vi "SVPO Average Dual-Channel Spectrum Measurements (Complex) with IC.vi"(0 "complex spectrum X":T9 {"spectrum info"."x-axis units" items=["Time (s)"=0, "Frequency-CB (Hz)"=1, "Frequency-CPB (Hz)"=1248, "Frequency-Arbitrary (Hz)"=2357, "Quefrency (s)"=2, "Revolutions (rev)"=3, "Order"=4, "Speed (RPM)"=11, "Speed (rad/s)"=21, "Index"=65535]; "spectrum info"."weighting filter" items=["Linear", "A-weighting", "B-weighting", "C-weighting", "ITU-R 468-4", "Dolby", "CCITT", "C-message", "Wb", "Wc", "Wd", "We", "Wf", "Wh", "Wj", "Wk", "Wm", "AES17 20 kHz lowpass", "AES17 40 kHz lowpass", "AES17 20 kHz highpass", "AES17 40 kHz highpass"]; "spectrum info"."dB reference [EU]" format="%.2f"; "spectrum info"."engineering units" items=["custom..."=0, "V"=1, "A"=21, "C"=30, "pC"=31, "s"=32, "-"=29, "Pa"=2, "N"=20, "g"=3, "m/s^2"=4, "m/s"=5, "m"=6, "mm/s"=12, "mm"=13, "micron/s"=14, "micron"=15, "in/s^2"=7, "in/s"=8, "in"=9, "mil/s"=10, "mil"=11, "rad/s^2"=16, "rad/s"=17, "rad"=18, "deg/s^2"=26, "deg/s"=27, "deg"=28, "RPM"=22, "cycle/s^2"=23, "Hz"=24, "cycle"=25, "strain"=19]; "spectrum info"."spectral info"."window" items=["None "=0, "Hanning"=1, "Hamming"=2, "Blackman-Harris"=3, "Exact Blackman"=4, "Blackman"=5, "Flat Top"=6, "4 Term B-Harris "=7, "7 Term B-Harris"=8, "Low Sidelobe"=9, "Force - Exponential"=10, "Gaussian"=62]}, 1 "complex spectrum Y":T9 {"spectrum info"."x-axis units" items=["Time (s)"=0, "Frequency-CB (Hz)"=1, "Frequency-CPB (Hz)"=1248, "Frequency-Arbitrary (Hz)"=2357, "Quefrency (s)"=2, "Revolutions (rev)"=3, "Order"=4, "Speed (RPM)"=11, "Speed (rad/s)"=21, "Index"=65535]; "spectrum info"."weighting filter" items=["Linear", "A-weighting", "B-weighting", "C-weighting", "ITU-R 468-4", "Dolby", "CCITT", "C-message", "Wb", "Wc", "Wd", "We", "Wf", "Wh", "Wj", "Wk", "Wm", "AES17 20 kHz lowpass", "AES17 40 kHz lowpass", "AES17 20 kHz highpass", "AES17 40 kHz highpass"]; "spectrum info"."dB reference [EU]" format="%.2f"; "spectrum info"."engineering units" items=["custom..."=0, "V"=1, "A"=21, "C"=30, "pC"=31, "s"=32, "-"=29, "Pa"=2, "N"=20, "g"=3, "m/s^2"=4, "m/s"=5, "m"=6, "mm/s"=12, "mm"=13, "micron/s"=14, "micron"=15, "in/s^2"=7, "in/s"=8, "in"=9, "mil/s"=10, "mil"=11, "rad/s^2"=16, "rad/s"=17, "rad"=18, "deg/s^2"=26, "deg/s"=27, "deg"=28, "RPM"=22, "cycle/s^2"=23, "Hz"=24, "cycle"=25, "strain"=19]; "spectrum info"."spectral info"."window" items=["None "=0, "Hanning"=1, "Hamming"=2, "Blackman-Harris"=3, "Exact Blackman"=4, "Blackman"=5, "Flat Top"=6, "4 Term B-Harris "=7, "7 Term B-Harris"=8, "Low Sidelobe"=9, "Force - Exponential"=10, "Gaussian"=62]}, 2 "averaging mode (RMS)":T1(ring)=enum."RMS averaging", 3 "averaging weighting mode (Linear)":enum16{"Linear", "Exponential"}(ring), 5 "initial conditions":T10 {"complex cross"."spectrum info"."x-axis units" items=["Time (s)"=0, "Frequency-CB (Hz)"=1, "Frequency-CPB (Hz)"=1248, "Frequency-Arbitrary (Hz)"=2357, "Quefrency (s)"=2, "Revolutions (rev)"=3, "Order"=4, "Speed (RPM)"=11, "Speed (rad/s)"=21, "Index"=65535]; "complex cross"."spectrum info"."weighting filter" items=["Linear", "A-weighting", "B-weighting", "C-weighting", "ITU-R 468-4", "Dolby", "CCITT", "C-message", "Wb", "Wc", "Wd", "We", "Wf", "Wh", "Wj", "Wk", "Wm", "AES17 20 kHz lowpass", "AES17 40 kHz lowpass", "AES17 20 kHz highpass", "AES17 40 kHz highpass"]; "complex cross"."spectrum info"."dB reference [EU]" format="%.2f"; "complex cross"."spectrum info"."engineering units" items=["custom..."=0, "V"=1, "A"=21, "C"=30, "pC"=31, "s"=32, "-"=29, "Pa"=2, "N"=20, "g"=3, "m/s^2"=4, "m/s"=5, "m"=6, "mm/s"=12, "mm"=13, "micron/s"=14, "micron"=15, "in/s^2"=7, "in/s"=8, "in"=9, "mil/s"=10, "mil"=11, "rad/s^2"=16, "rad/s"=17, "rad"=18, "deg/s^2"=26, "deg/s"=27, "deg"=28, "RPM"=22, "cycle/s^2"=23, "Hz"=24, "cycle"=25, "strain"=19]; "complex cross"."spectrum info"."spectral info"."window" items=["None "=0, "Hanning"=1, "Hamming"=2, "Blackman-Harris"=3, "Exact Blackman"=4, "Blackman"=5, "Flat Top"=6, "4 Term B-Harris "=7, "7 Term B-Harris"=8, "Low Sidelobe"=9, "Force - Exponential"=10, "Gaussian"=62]; "complex X"."spectrum info"."x-axis units" items=["Time (s)"=0, "Frequency-CB (Hz)"=1, "Frequency-CPB (Hz)"=1248, "Frequency-Arbitrary (Hz)"=2357, "Quefrency (s)"=2, "Revolutions (rev)"=3, "Order"=4, "Speed (RPM)"=11, "Speed (rad/s)"=21, "Index"=65535]; "complex X"."spectrum info"."weighting filter" items=["Linear", "A-weighting", "B-weighting", "C-weighting", "ITU-R 468-4", "Dolby", "CCITT", "C-message", "Wb", "Wc", "Wd", "We", "Wf", "Wh", "Wj", "Wk", "Wm", "AES17 20 kHz lowpass", "AES17 40 kHz lowpass", "AES17 20 kHz highpass", "AES17 40 kHz highpass"]; "complex X"."spectrum info"."dB reference [EU]" format="%.2f"; "complex X"."spectrum info"."engineering units" items=["custom..."=0, "V"=1, "A"=21, "C"=30, "pC"=31, "s"=32, "-"=29, "Pa"=2, "N"=20, "g"=3, "m/s^2"=4, "m/s"=5, "m"=6, "mm/s"=12, "mm"=13, "micron/s"=14, "micron"=15, "in/s^2"=7, "in/s"=8, "in"=9, "mil/s"=10, "mil"=11, "rad/s^2"=16, "rad/s"=17, "rad"=18, "deg/s^2"=26, "deg/s"=27, "deg"=28, "RPM"=22, "cycle/s^2"=23, "Hz"=24, "cycle"=25, "strain"=19]; "complex X"."spectrum info"."spectral info"."window" items=["None "=0, "Hanning"=1, "Hamming"=2, "Blackman-Harris"=3, "Exact Blackman"=4, "Blackman"=5, "Flat Top"=6, "4 Term B-Harris "=7, "7 Term B-Harris"=8, "Low Sidelobe"=9, "Force - Exponential"=10, "Gaussian"=62]; "complex Y"."spectrum info"."x-axis units" items=["Time (s)"=0, "Frequency-CB (Hz)"=1, "Frequency-CPB (Hz)"=1248, "Frequency-Arbitrary (Hz)"=2357, "Quefrency (s)"=2, "Revolutions (rev)"=3, "Order"=4, "Speed (RPM)"=11, "Speed (rad/s)"=21, "Index"=65535]; "complex Y"."spectrum info"."weighting filter" items=["Linear", "A-weighting", "B-weighting", "C-weighting", "ITU-R 468-4", "Dolby", "CCITT", "C-message", "Wb", "Wc", "Wd", "We", "Wf", "Wh", "Wj", "Wk", "Wm", "AES17 20 kHz lowpass", "AES17 40 kHz lowpass", "AES17 20 kHz highpass", "AES17 40 kHz highpass"]; "complex Y"."spectrum info"."dB reference [EU]" format="%.2f"; "complex Y"."spectrum info"."engineering units" items=["custom..."=0, "V"=1, "A"=21, "C"=30, "pC"=31, "s"=32, "-"=29, "Pa"=2, "N"=20, "g"=3, "m/s^2"=4, "m/s"=5, "m"=6, "mm/s"=12, "mm"=13, "micron/s"=14, "micron"=15, "in/s^2"=7, "in/s"=8, "in"=9, "mil/s"=10, "mil"=11, "rad/s^2"=16, "rad/s"=17, "rad"=18, "deg/s^2"=26, "deg/s"=27, "deg"=28, "RPM"=22, "cycle/s^2"=23, "Hz"=24, "cycle"=25, "strain"=19]; "complex Y"."spectrum info"."spectral info"."window" items=["None "=0, "Hanning"=1, "Hamming"=2, "Blackman-Harris"=3, "Exact Blackman"=4, "Blackman"=5, "Flat Top"=6, "4 Term B-Harris "=7, "7 Term B-Harris"=8, "Low Sidelobe"=9, "Force - Exponential"=10, "Gaussian"=62]}, 6 "exponential weight (10 %)":dbl=10.0 min=0.0 max=100.0 step=5.0, 8 "measurement (Cross)":T2(ring), 9 "restart averaging (F)":bool) -> (12 "coherence":cluster{"f0":dbl, "df":dbl, "coherence":dbl[]}, 13 "averages completed out":dbl=1.0, 14 "average measurement spectrum out":T9 {"spectrum info"."x-axis units" items=["Time (s)"=0, "Frequency-CB (Hz)"=1, "Frequency-CPB (Hz)"=1248, "Frequency-Arbitrary (Hz)"=2357, "Quefrency (s)"=2, "Revolutions (rev)"=3, "Order"=4, "Speed (RPM)"=11, "Speed (rad/s)"=21, "Index"=65535]; "spectrum info"."weighting filter" items=["Linear", "A-weighting", "B-weighting", "C-weighting", "ITU-R 468-4", "Dolby", "CCITT", "C-message", "Wb", "Wc", "Wd", "We", "Wf", "Wh", "Wj", "Wk", "Wm", "AES17 20 kHz lowpass", "AES17 40 kHz lowpass", "AES17 20 kHz highpass", "AES17 40 kHz highpass"]; "spectrum info"."dB reference [EU]" format="%.2f"; "spectrum info"."engineering units" items=["custom..."=0, "V"=1, "A"=21, "C"=30, "pC"=31, "s"=32, "-"=29, "Pa"=2, "N"=20, "g"=3, "m/s^2"=4, "m/s"=5, "m"=6, "mm/s"=12, "mm"=13, "micron/s"=14, "micron"=15, "in/s^2"=7, "in/s"=8, "in"=9, "mil/s"=10, "mil"=11, "rad/s^2"=16, "rad/s"=17, "rad"=18, "deg/s^2"=26, "deg/s"=27, "deg"=28, "RPM"=22, "cycle/s^2"=23, "Hz"=24, "cycle"=25, "strain"=19]; "spectrum info"."spectral info"."window" items=["None "=0, "Hanning"=1, "Hamming"=2, "Blackman-Harris"=3, "Exact Blackman"=4, "Blackman"=5, "Flat Top"=6, "4 Term B-Harris "=7, "7 Term B-Harris"=8, "Low Sidelobe"=9, "Force - Exponential"=10, "Gaussian"=62]}, 19 "final conditions":T10 {"complex cross"."spectrum info"."x-axis units" items=["Time (s)"=0, "Frequency-CB (Hz)"=1, "Frequency-CPB (Hz)"=1248, "Frequency-Arbitrary (Hz)"=2357, "Quefrency (s)"=2, "Revolutions (rev)"=3, "Order"=4, "Speed (RPM)"=11, "Speed (rad/s)"=21, "Index"=65535]; "complex cross"."spectrum info"."weighting filter" items=["Linear", "A-weighting", "B-weighting", "C-weighting", "ITU-R 468-4", "Dolby", "CCITT", "C-message", "Wb", "Wc", "Wd", "We", "Wf", "Wh", "Wj", "Wk", "Wm", "AES17 20 kHz lowpass", "AES17 40 kHz lowpass", "AES17 20 kHz highpass", "AES17 40 kHz highpass"]; "complex cross"."spectrum info"."dB reference [EU]" format="%.2f"; "complex cross"."spectrum info"."engineering units" items=["custom..."=0, "V"=1, "A"=21, "C"=30, "pC"=31, "s"=32, "-"=29, "Pa"=2, "N"=20, "g"=3, "m/s^2"=4, "m/s"=5, "m"=6, "mm/s"=12, "mm"=13, "micron/s"=14, "micron"=15, "in/s^2"=7, "in/s"=8, "in"=9, "mil/s"=10, "mil"=11, "rad/s^2"=16, "rad/s"=17, "rad"=18, "deg/s^2"=26, "deg/s"=27, "deg"=28, "RPM"=22, "cycle/s^2"=23, "Hz"=24, "cycle"=25, "strain"=19]; "complex cross"."spectrum info"."spectral info"."window" items=["None "=0, "Hanning"=1, "Hamming"=2, "Blackman-Harris"=3, "Exact Blackman"=4, "Blackman"=5, "Flat Top"=6, "4 Term B-Harris "=7, "7 Term B-Harris"=8, "Low Sidelobe"=9, "Force - Exponential"=10, "Gaussian"=62]; "complex X"."spectrum info"."x-axis units" items=["Time (s)"=0, "Frequency-CB (Hz)"=1, "Frequency-CPB (Hz)"=1248, "Frequency-Arbitrary (Hz)"=2357, "Quefrency (s)"=2, "Revolutions (rev)"=3, "Order"=4, "Speed (RPM)"=11, "Speed (rad/s)"=21, "Index"=65535]; "complex X"."spectrum info"."weighting filter" items=["Linear", "A-weighting", "B-weighting", "C-weighting", "ITU-R 468-4", "Dolby", "CCITT", "C-message", "Wb", "Wc", "Wd", "We", "Wf", "Wh", "Wj", "Wk", "Wm", "AES17 20 kHz lowpass", "AES17 40 kHz lowpass", "AES17 20 kHz highpass", "AES17 40 kHz highpass"]; "complex X"."spectrum info"."dB reference [EU]" format="%.2f"; "complex X"."spectrum info"."engineering units" items=["custom..."=0, "V"=1, "A"=21, "C"=30, "pC"=31, "s"=32, "-"=29, "Pa"=2, "N"=20, "g"=3, "m/s^2"=4, "m/s"=5, "m"=6, "mm/s"=12, "mm"=13, "micron/s"=14, "micron"=15, "in/s^2"=7, "in/s"=8, "in"=9, "mil/s"=10, "mil"=11, "rad/s^2"=16, "rad/s"=17, "rad"=18, "deg/s^2"=26, "deg/s"=27, "deg"=28, "RPM"=22, "cycle/s^2"=23, "Hz"=24, "cycle"=25, "strain"=19]; "complex X"."spectrum info"."spectral info"."window" items=["None "=0, "Hanning"=1, "Hamming"=2, "Blackman-Harris"=3, "Exact Blackman"=4, "Blackman"=5, "Flat Top"=6, "4 Term B-Harris "=7, "7 Term B-Harris"=8, "Low Sidelobe"=9, "Force - Exponential"=10, "Gaussian"=62]; "complex Y"."spectrum info"."x-axis units" items=["Time (s)"=0, "Frequency-CB (Hz)"=1, "Frequency-CPB (Hz)"=1248, "Frequency-Arbitrary (Hz)"=2357, "Quefrency (s)"=2, "Revolutions (rev)"=3, "Order"=4, "Speed (RPM)"=11, "Speed (rad/s)"=21, "Index"=65535]; "complex Y"."spectrum info"."weighting filter" items=["Linear", "A-weighting", "B-weighting", "C-weighting", "ITU-R 468-4", "Dolby", "CCITT", "C-message", "Wb", "Wc", "Wd", "We", "Wf", "Wh", "Wj", "Wk", "Wm", "AES17 20 kHz lowpass", "AES17 40 kHz lowpass", "AES17 20 kHz highpass", "AES17 40 kHz highpass"]; "complex Y"."spectrum info"."dB reference [EU]" format="%.2f"; "complex Y"."spectrum info"."engineering units" items=["custom..."=0, "V"=1, "A"=21, "C"=30, "pC"=31, "s"=32, "-"=29, "Pa"=2, "N"=20, "g"=3, "m/s^2"=4, "m/s"=5, "m"=6, "mm/s"=12, "mm"=13, "micron/s"=14, "micron"=15, "in/s^2"=7, "in/s"=8, "in"=9, "mil/s"=10, "mil"=11, "rad/s^2"=16, "rad/s"=17, "rad"=18, "deg/s^2"=26, "deg/s"=27, "deg"=28, "RPM"=22, "cycle/s^2"=23, "Hz"=24, "cycle"=25, "strain"=19]; "complex Y"."spectrum info"."spectral info"."window" items=["None "=0, "Hanning"=1, "Hamming"=2, "Blackman-Harris"=3, "Exact Blackman"=4, "Blackman"=5, "Flat Top"=6, "4 Term B-Harris "=7, "7 Term B-Harris"=8, "Low Sidelobe"=9, "Force - Exponential"=10, "Gaussian"=62]})   [LabVIEW 2017]
doc: "Measures the frequency response of the input signals and the coherence based on the current and previous input signals. This VI returns results such as <B>Magnitude</B>, <B>Phase</B>, <B>Coherence</B>, <B>Real</B>, and <B>Imaginary</B>."
uses:
  <vilib>/addons/_NISVFA/_Shared subVIs/Controls/svc_Dual CH Spectral Measurements Avg State.ctl
  <vilib>/addons/_NISVFA/_Shared subVIs/Controls/svc_Spectrum Info.ctl
  <vilib>/addons/_NISVFA/_Shared subVIs/Controls/svc_X-Axis Units.ctl
  <vilib>/addons/_NISVFA/_Shared subVIs/Controls/svc_Spectrum Type.ctl
  <vilib>/addons/_NISVFA/_Shared subVIs/Controls/svc_Engineering Units Text Ring.ctl
  <vilib>/addons/_NISVFA/_Shared subVIs/Controls/svc_Weighting Filter Text Ring.ctl
  <vilib>/addons/_NISVFA/_Shared subVIs/Controls/svc_Complimentary Spectrum Units.ctl
  <vilib>/addons/_NISVFA/_Shared subVIs/Common/sv_Get NI Property Name String.vi
  <vilib>/addons/_NISVFA/_Shared subVIs/Spectrum Averaging/svpo_Average Array (complex).vi
  <vilib>/addons/_NISVFA/_Shared subVIs/Spectrum Info/svfa_Get Averaging Mode from Spectrum Info.vi
  <vilib>/addons/_NISVFA/_Shared subVIs/Spectrum Averaging/svpo_Average Array (real).vi
  <vilib>/addons/_NISVFA/_Shared subVIs/Spectrum Info/sfva_Set SV Info in Spectrum Info Description.vi
  <vilib>/addons/_NISVFA/_Shared subVIs/Spectrum Info/sfva_Get SV Info from Spectrum Info Description.vi
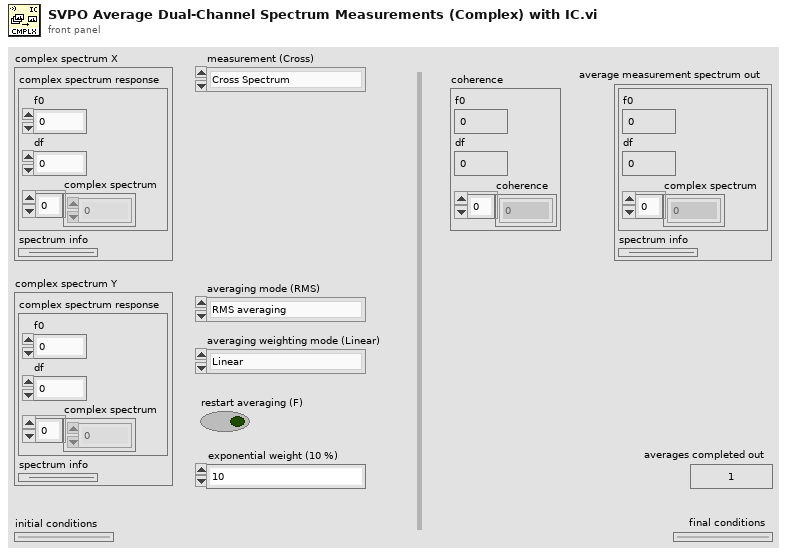
[diagram p1: front panel]
types:
  T1 = enum16{"No averaging", "Vector averaging", "RMS averaging"}
  T2 = enum16{"Cross Spectrum", "Frequency Response (H1)", "Frequency Response (H2)", "Frequency Response (H3)"}
  T3 = typedef "svc_Spectrum Info.ctl" = cluster{"channel name":string, "description":string, "x-axis units":T4, "spectral info":cluster{"spectrum type":T5, "linear/dB":enum16{"linear", "dB"}, "window":u16, "window size":i32, "FFT size":i32}, "engineering units":T6, "custom label":string, "dB reference [EU]":dbl, "peak units":enum16{"rms", "peak", "peak-peak"}, "weighting filter":T7, "spectral density?":bool, "unit label":string, "spectrum skewed?":bool, "complimentary spectrum units":T8}
  T4 = typedef "svc_X-Axis Units.ctl" = u16
  T5 = typedef "svc_Spectrum Type.ctl" = enum16{"FFT Spectrum [complex]", "Amplitude [Magnitude]", "Power [Magnitude^2]", "Cross Spectrum [complex]", "Frequency Response [Complex]"}
  T6 = typedef "svc_Engineering Units Text Ring.ctl" = u16
  T7 = typedef "svc_Weighting Filter Text Ring.ctl" = u16
  T8 = typedef "svc_Complimentary Spectrum Units.ctl" = enum16{"none", "radians", "degrees", "cycles", "imaginary"}
  T9 = cluster{"complex spectrum response":cluster{"f0":dbl, "df":dbl, "complex spectrum":cdb[]}, "spectrum info":T3}
  T10 = typedef "svc_Dual CH Spectral Measurements Avg State.ctl" = cluster{"Real X^2":cluster{"f0":dbl, "df":dbl, "X^2":dbl[]}, "Real Y^2":cluster{"f0":dbl, "df":dbl, "Y^2":dbl[]}, "complex cross":cluster{"complex spectrum response":cluster{"f0":dbl, "df":dbl, "X*Y":cdb[]}, "spectrum info":T3}, "complex X":cluster{"complex spectrum response":cluster{"f0":dbl, "df":dbl, "complex X":cdb[]}, "spectrum info":T3}, "complex Y":cluster{"complex spectrum response":cluster{"f0":dbl, "df":dbl, "complex Y":cdb[]}, "spectrum info":T3}, "averages completed":dbl}
  T11 = enum16{"No averaging", "Vector averaging", "RMS averaging", "Peak hold"}
  T12 = cluster{"complex spectrum response":cluster{"f0":dbl, "df":dbl, "X*Y":cdb[]}, "spectrum info":T3}
  T13 = cluster{"complex spectrum response":cluster{"f0":dbl, "df":dbl, "complex X":cdb[]}, "spectrum info":T3}
  T14 = cluster{"complex spectrum response":cluster{"f0":dbl, "df":dbl, "complex Y":cdb[]}, "spectrum info":T3}
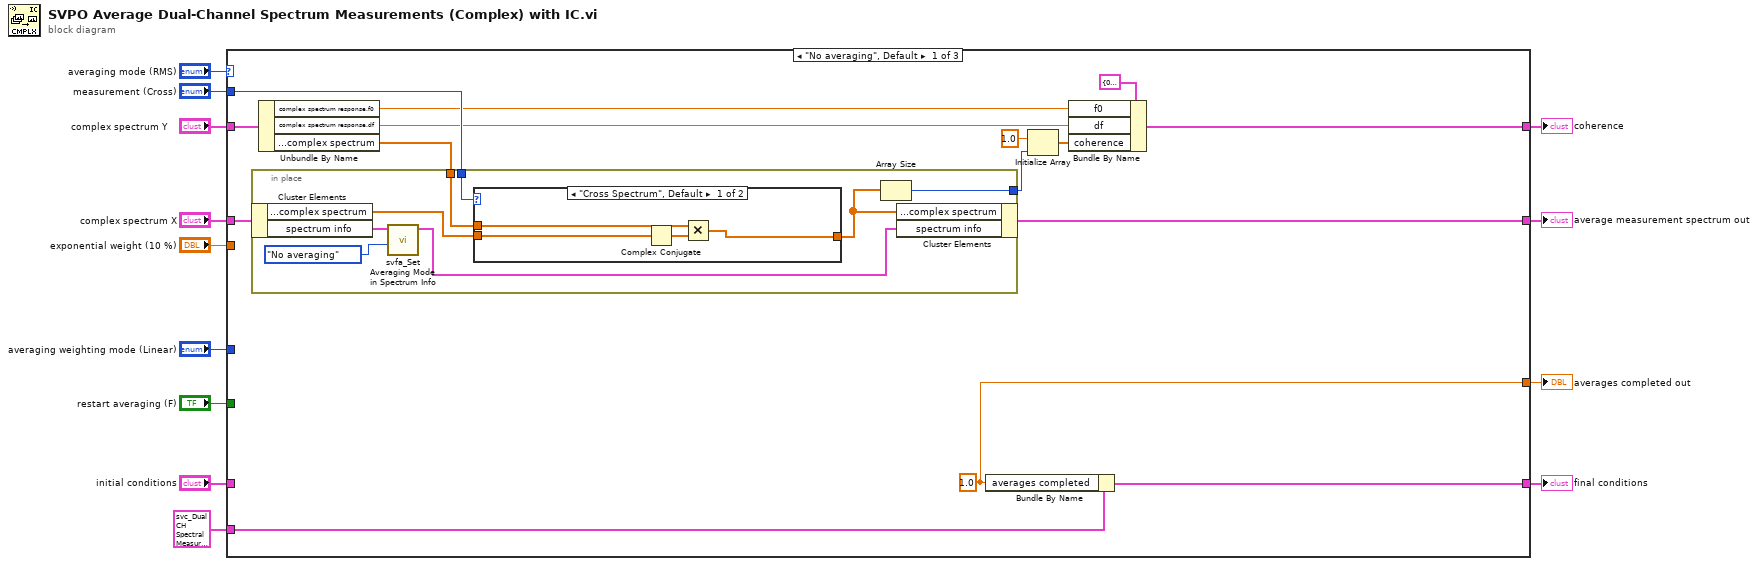
[diagram p0: block diagram]
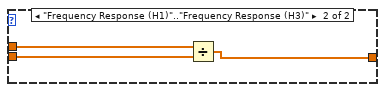
[diagram p2: hidden frame]
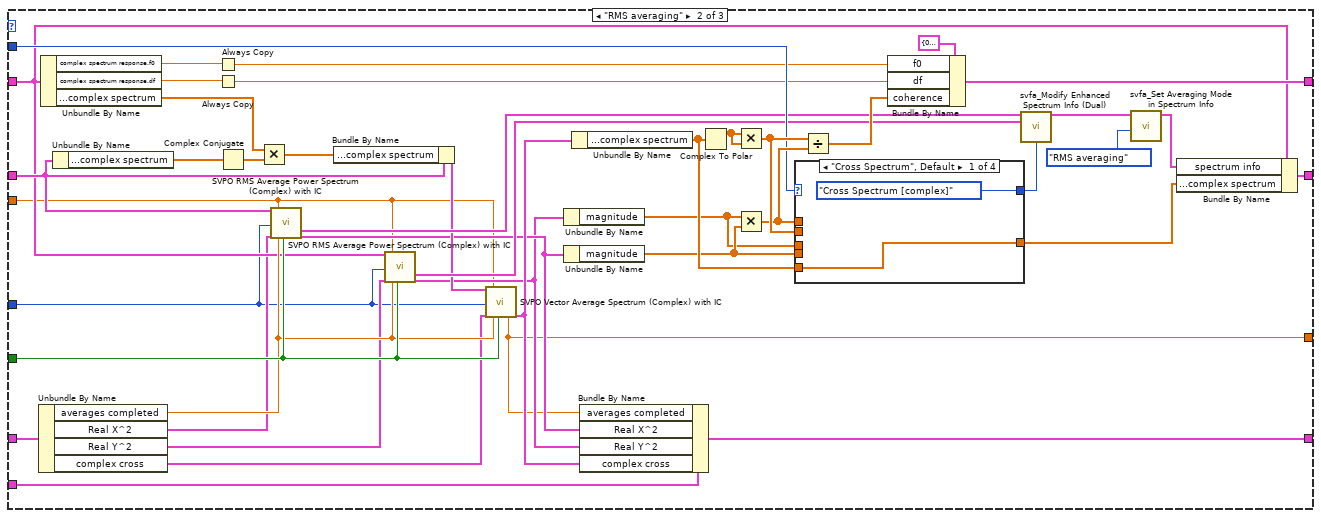
[diagram p3: hidden frame]
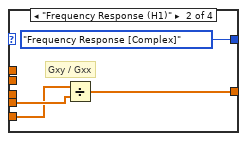
[diagram p4: hidden frame]
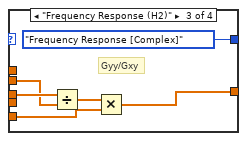
[diagram p5: hidden frame]
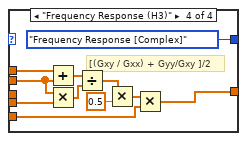
[diagram p6: hidden frame]
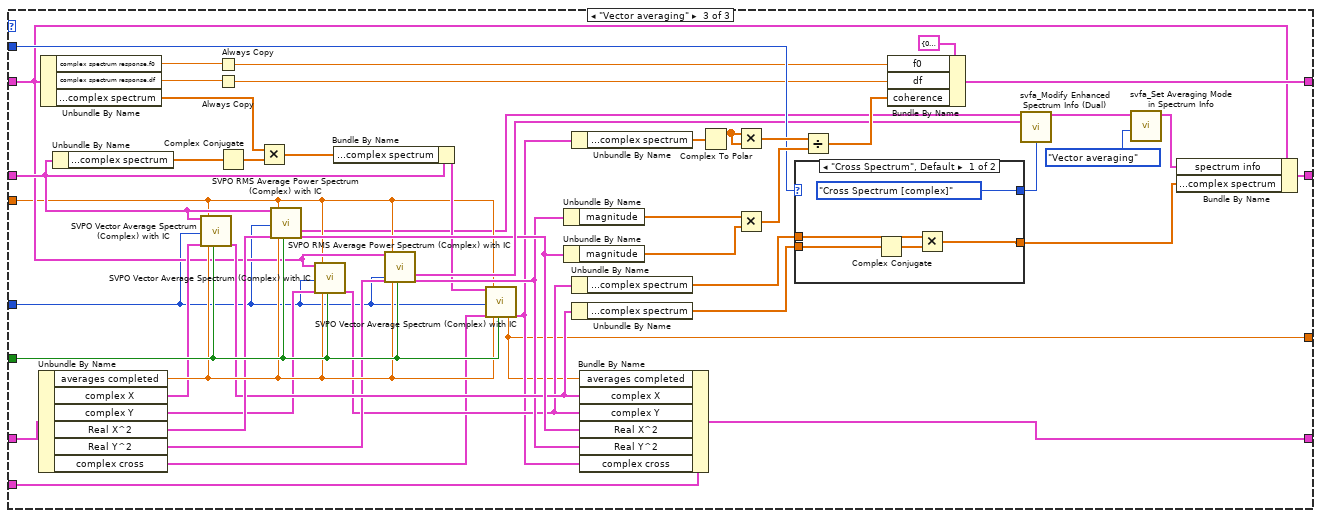
[diagram p7: hidden frame]
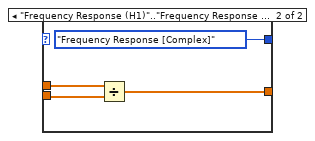
[diagram p8: hidden frame]
diagram:
  n1 = case shown="\"No averaging\", Default" "averaging mode (RMS)" {
    tunnel: "measurement (Cross)" -> [w28 w68 w140]
    tunnel: "complex spectrum Y" -> [w27 w54 w122]
    tunnel: "complex spectrum X" -> [w15 w55 w127]
    tunnel: [w14 w66 w138] -> w6
    tunnel: "restart averaging (F)" -> [_ w64 w133]
    tunnel: "averaging weighting mode (Linear)" -> [_ w48 w115]
    tunnel: "exponential weight (10 %)" -> [_ w47 w114]
    tunnel: [w21 w80 w152] -> w10
    tunnel: [w18 w77 w149] -> w11
    tunnel: "initial conditions" -> [_ w76 w148]
    tunnel: T10 {"Real X^2"={"f0"=0.0, "df"=0.0, "X^2"=[]}, "Real Y^2"={"f0"=0.0, "df"=0.0, "Y^2"=[]}, "complex cross"={"complex spectrum response"={"f0"=0.0, "df"=0.0, "X*Y"=[]}, "spectrum info"={"channel name"="", "description"="", "x-axis units"=0, "spectral info"={"spectrum type"=enum."FFT Spectrum [complex]", "linear/dB"=enum."linear", "window"=0, "window size"=0, "FFT size"=0}, "engineering units"=0, "custom label"="", "dB reference [EU]"=0.0, "peak units"=enum."rms", "weighting filter"=0, "spectral density?"=FALSE, "unit label"="", "spectrum skewed?"=FALSE, "complimentary spectrum units"=enum."none"}}, "complex X"={"complex spectrum response"={"f0"=0.0, "df"=0.0, "complex X"=[]}, "spectrum info"={"channel name"="", "description"="", "x-axis units"=0, "spectral info"={"spectrum type"=enum."FFT Spectrum [complex]", "linear/dB"=enum."linear", "window"=0, "window size"=0, "FFT size"=0}, "engineering units"=0, "custom label"="", "dB reference [EU]"=0.0, "peak units"=enum."rms", "weighting filter"=0, "spectral density?"=FALSE, "unit label"="", "spectrum skewed?"=FALSE, "complimentary spectrum units"=enum."none"}}, "complex Y"={"complex spectrum response"={"f0"=0.0, "df"=0.0, "complex Y"=[]}, "spectrum info"={"channel name"="", "description"="", "x-axis units"=0, "spectral info"={"spectrum type"=enum."FFT Spectrum [complex]", "linear/dB"=enum."linear", "window"=0, "window size"=0, "FFT size"=0}, "engineering units"=0, "custom label"="", "dB reference [EU]"=0.0, "peak units"=enum."rms", "weighting filter"=0, "spectral density?"=FALSE, "unit label"="", "spectrum skewed?"=FALSE, "complimentary spectrum units"=enum."none"}}, "averages completed"=0.0} -> [w19 w78 w150]
    tunnel: [w17 w49 w116] -> w1
    frame "No averaging", Default {
      w17 = 1.0 ("averages completed")
      n2 = Unbundle By Name(w27) -> ("complex spectrum response.f0"=w25:dbl, "complex spectrum response.df"=w24:dbl, "complex spectrum response.complex spectrum"=w26:cdb[])
      n3 = in-place {
        in-place-border: w28 -> [w36]
        in-place-border: w26 -> [w35]
        in-place-border: [w32] -> w16
        n4 = in-place-cluster #1(w15) -> ("complex spectrum response.complex spectrum"=w34:cdb[], "spectrum info"=w30:T3)
        n5 = call <vilib>:"svfa_Set Averaging Mode in Spectrum Info.vi"("averaging mode"=T11."No averaging", "spectrum info in"=w30) -> ("spectrum info out"=w29:T3)  [unwired: 8 in, 1 out]
        n6 = case shown="\"Cross Spectrum\", Default" w36 {
          tunnel: w35 -> [w37 w43]
          tunnel: w34 -> [w38 w42]
          tunnel: [w39 w41] -> w33
          frame "Cross Spectrum", Default {
            n7 = Complex Conjugate(1:w38) -> (0:w40:cdb[])
            n8 = Multiply(x=w37, y=w40) -> (x*y=w39:cdb[])
          }
          frame "Frequency Response (H1)".."Frequency Response (H3)" {
            n9 = Divide(x=w43, y=w42) -> (x/y=w41:cdb[])
          }
        }
        n10 = Array Size(array=w33) -> (size(s)=w32:i32)
        n11 = in-place-cluster #1("complex spectrum response.complex spectrum"=w33, "spectrum info"=w29) -> (w14:T9)
      }
      n12 = Bundle By Name(cluster=w19, "averages completed"=w17) -> (w18:T10)
      n13 = Initialize Array(1.0 ("element"), w16) -> (w22:dbl[])
      n14 = Bundle By Name(cluster=cluster{"f0":dbl, "df":dbl, "coherence":dbl[]} {"f0"=0.0, "df"=0.0, "coherence"=[]} ("coherence"), "f0"=w25, "df"=w24, "coherence"=w22) -> (w21:cluster{"f0":dbl, "df":dbl, "coherence":dbl[]})
    }
    frame "RMS averaging" {
      n15 = Unbundle By Name(w76) -> ("averages completed"=w59:dbl, "Real X^2"=w52:cluster{"f0":dbl, "df":dbl, "X^2":dbl[]}, "Real Y^2"=w51:cluster{"f0":dbl, "df":dbl, "Y^2":dbl[]}, "complex cross"=w50:T12)
      n16 = Unbundle By Name(w54) -> ("complex spectrum response.f0"=w82:dbl, "complex spectrum response.df"=w81:dbl, "complex spectrum response.complex spectrum"=w86:cdb[])
      n17 = Unbundle By Name(w55) -> ("complex spectrum response.complex spectrum"=w85:cdb[])
      n18 = Always Copy(1:w82) -> (0:w61:dbl)
      n19 = Always Copy(1:w81) -> (0:w60:dbl)
      n20 = Complex Conjugate(1:w85) -> (0:w79:cdb[])
      n21 = Multiply(x=w86, y=w79) -> (x*y=w84:cdb[])
      n22 = call <vilib>:"SVPO RMS Average Power Spectrum (Complex) with IC.vi"("complex spectrum [EU rms]"=w55, "averaging weighting mode"=w48, "average power spectrum in"=w52, "exponential weight (10 %)"=w47, "averages completed in"=w59, "restart averaging (F)"=w64) -> ("spectrum info"=w62:T3, "average power spectrum out"=w56:cluster{"f0":dbl, "df":dbl, "magnitude":dbl[]})  [unwired: 11 in, 1 out]
      n23 = Bundle By Name(cluster=w55, "complex spectrum response.complex spectrum"=w84) -> (w57:T9)
      n24 = call <vilib>:"SVPO RMS Average Power Spectrum (Complex) with IC.vi"("complex spectrum [EU rms]"=w54, "averaging weighting mode"=w48, "average power spectrum in"=w51, "exponential weight (10 %)"=w47, "averages completed in"=w59, "restart averaging (F)"=w64) -> ("spectrum info"=w63:T3, "average power spectrum out"=w53:cluster{"f0":dbl, "df":dbl, "magnitude":dbl[]})  [unwired: 11 in, 1 out]
      n25 = call <vilib>:"SVPO Vector Average Spectrum (Complex) with IC.vi"("complex spectrum [EU rms]"=w57, "averaging weighting mode"=w48, "average complex spectrum in"=w50, "exponential weight (10 %)"=w47, "averages completed in"=w59, "restart averaging (F)"=w64) -> ("averages completed out"=w49:dbl, "average complex spectrum out"=w58:T9)  [unwired: 12 in]
      n26 = Unbundle By Name(w53) -> ("magnitude"=w71:dbl[])
      n27 = Unbundle By Name(w56) -> ("magnitude"=w72:dbl[])
      n28 = Unbundle By Name(w58) -> ("complex spectrum response.complex spectrum"=w73:cdb[])
      n29 = Bundle By Name(cluster=w78, "averages completed"=w49, "Real X^2"=w56, "Real Y^2"=w53, "complex cross"=w58) -> (w77:T10)
      n30 = Complex To Polar(r * e^(i*theta)=w73) -> (r=w75:dbl[])  [unwired: 1 out]
      n31 = Multiply(x=w75, y=w75) -> (x*y=w70:dbl[])
      n32 = Multiply(x=w71, y=w72) -> (x*y=w69:dbl[])
      n33 = case shown="\"Cross Spectrum\", Default" w68 {
        tunnel: [w88 w92 w94 w107] -> w67
        tunnel: w72 -> [_ w91 _ w103]
        tunnel: w71 -> [_ _ w98 _]
        tunnel: w73 -> [w88 w90 w95 w100]
        tunnel: w70 -> [_ _ w97 w101]
        tunnel: w69 -> [_ _ _ w106]
        tunnel: [svc_Spectrum_Type."Cross Spectrum [complex]" ("spectrum type") svc_Spectrum_Type."Frequency Response [Complex]" ("spectrum type") svc_Spectrum_Type."Frequency Response [Complex]" ("spectrum type") svc_Spectrum_Type."Frequency Response [Complex]" ("spectrum type")] -> w65
        frame "Cross Spectrum", Default {
        }
        frame "Frequency Response (H1)" {
          # "Gxy / Gxx"
          n34 = Divide(x=w90, y=w91) -> (x/y=w92:cdb[])
        }
        frame "Frequency Response (H2)" {
          # "Gyy/Gxy"
          n35 = Divide(x=w98, y=w97) -> (x/y=w96:dbl[])
          n36 = Multiply(x=w96, y=w95) -> (x*y=w94:cdb[])
        }
        frame "Frequency Response (H3)" {
          # "[(Gxy / Gxx) + Gyy/Gxy ]/2"
          n37 = Add(x=w106, y=w101) -> (x+y=w105:dbl[])
          n38 = Multiply(x=w101, y=w103) -> (x*y=w102:dbl[])
          n39 = Divide(x=w105, y=w102) -> (x/y=w104:dbl[])
          n40 = Multiply(x=w104, y=0.5) -> (x*y=w108:dbl[])
          n41 = Multiply(x=w108, y=w100) -> (x*y=w107:cdb[])
        }
      }
      n42 = Divide(x=w70, y=w69) -> (x/y=w74:dbl[])
      n43 = Bundle By Name(cluster=cluster{"f0":dbl, "df":dbl, "coherence":dbl[]} {"f0"=0.0, "df"=0.0, "coherence"=[]} ("coherence"), "f0"=w61, "df"=w60, "coherence"=w74) -> (w80:cluster{"f0":dbl, "df":dbl, "coherence":dbl[]})
      n44 = call <vilib>:"svfa_Modify Enhanced Spectrum Info (Dual).vi"("spectrum info X"=w62, "spectrum info Y"=w63, "spectrum type"=w65) -> ("spectrum info"=w46:T3)  [unwired: 10 in, 2 out]
      n45 = call <vilib>:"svfa_Set Averaging Mode in Spectrum Info.vi"("averaging mode"=T11."RMS averaging", "spectrum info in"=w46) -> ("spectrum info out"=w45:T3)  [unwired: 8 in, 1 out]
      n46 = Bundle By Name(cluster=w54, "spectrum info"=w45, "complex spectrum response.complex spectrum"=w67) -> (w66:T9)
    }
    frame "Vector averaging" {
      n47 = Unbundle By Name(w148) -> ("averages completed"=w130:dbl, "complex X"=w129:T13, "complex Y"=w124:T14, "Real X^2"=w128:cluster{"f0":dbl, "df":dbl, "X^2":dbl[]}, "Real Y^2"=w123:cluster{"f0":dbl, "df":dbl, "Y^2":dbl[]}, "complex cross"=w118:T12)
      n48 = Unbundle By Name(w122) -> ("complex spectrum response.f0"=w154:dbl, "complex spectrum response.df"=w153:dbl, "complex spectrum response.complex spectrum"=w158:cdb[])
      n49 = Unbundle By Name(w127) -> ("complex spectrum response.complex spectrum"=w157:cdb[])
      n50 = call <vilib>:"SVPO Vector Average Spectrum (Complex) with IC.vi"("complex spectrum [EU rms]"=w127, "averaging weighting mode"=w115, "average complex spectrum in"=w129, "exponential weight (10 %)"=w114, "averages completed in"=w130, "restart averaging (F)"=w133) -> ("average complex spectrum out"=w125:T9)  [unwired: 12 in, 1 out]
      n51 = Always Copy(1:w154) -> (0:w135:dbl)
      n52 = Always Copy(1:w153) -> (0:w134:dbl)
      n53 = Complex Conjugate(1:w157) -> (0:w151:cdb[])
      n54 = Multiply(x=w158, y=w151) -> (x*y=w156:cdb[])
      n55 = call <vilib>:"SVPO RMS Average Power Spectrum (Complex) with IC.vi"("complex spectrum [EU rms]"=w127, "averaging weighting mode"=w115, "average power spectrum in"=w128, "exponential weight (10 %)"=w114, "averages completed in"=w130, "restart averaging (F)"=w133) -> ("spectrum info"=w113:T3, "average power spectrum out"=w126:cluster{"f0":dbl, "df":dbl, "magnitude":dbl[]})  [unwired: 11 in, 1 out]
      n56 = call <vilib>:"SVPO Vector Average Spectrum (Complex) with IC.vi"("complex spectrum [EU rms]"=w122, "averaging weighting mode"=w115, "average complex spectrum in"=w124, "exponential weight (10 %)"=w114, "averages completed in"=w130, "restart averaging (F)"=w133) -> ("average complex spectrum out"=w120:T9)  [unwired: 12 in, 1 out]
      n57 = Bundle By Name(cluster=w127, "complex spectrum response.complex spectrum"=w156) -> (w117:T9)
      n58 = call <vilib>:"SVPO RMS Average Power Spectrum (Complex) with IC.vi"("complex spectrum [EU rms]"=w122, "averaging weighting mode"=w115, "average power spectrum in"=w123, "exponential weight (10 %)"=w114, "averages completed in"=w130, "restart averaging (F)"=w133) -> ("spectrum info"=w136:T3, "average power spectrum out"=w121:cluster{"f0":dbl, "df":dbl, "magnitude":dbl[]})  [unwired: 11 in, 1 out]
      n59 = call <vilib>:"SVPO Vector Average Spectrum (Complex) with IC.vi"("complex spectrum [EU rms]"=w117, "averaging weighting mode"=w115, "average complex spectrum in"=w118, "exponential weight (10 %)"=w114, "averages completed in"=w130, "restart averaging (F)"=w133) -> ("averages completed out"=w116:dbl, "average complex spectrum out"=w119:T9)  [unwired: 12 in]
      n60 = Unbundle By Name(w121) -> ("magnitude"=w143:dbl[])
      n61 = Unbundle By Name(w126) -> ("magnitude"=w144:dbl[])
      n62 = Unbundle By Name(w119) -> ("complex spectrum response.complex spectrum"=w145:cdb[])
      n63 = Unbundle By Name(w120) -> ("complex spectrum response.complex spectrum"=w131:cdb[])
      n64 = Unbundle By Name(w125) -> ("complex spectrum response.complex spectrum"=w132:cdb[])
      n65 = Bundle By Name(cluster=w150, "averages completed"=w116, "complex X"=w125, "complex Y"=w120, "Real X^2"=w126, "Real Y^2"=w121, "complex cross"=w119) -> (w149:T10)
      n66 = Complex To Polar(r * e^(i*theta)=w145) -> (r=w147:dbl[])  [unwired: 1 out]
      n67 = Multiply(x=w147, y=w147) -> (x*y=w142:dbl[])
      n68 = Multiply(x=w143, y=w144) -> (x*y=w141:dbl[])
      n69 = case shown="\"Cross Spectrum\", Default" w140 {
        tunnel: [w159 w167] -> w139
        tunnel: [svc_Spectrum_Type."Cross Spectrum [complex]" ("spectrum type") svc_Spectrum_Type."Frequency Response [Complex]" ("spectrum type")] -> w137
        tunnel: w132 -> [w161 w164]
        tunnel: w131 -> [w160 w165]
        frame "Cross Spectrum", Default {
          n70 = Complex Conjugate(1:w161) -> (0:w162:cdb[])
          n71 = Multiply(x=w160, y=w162) -> (x*y=w159:cdb[])
        }
        frame "Frequency Response (H1)".."Frequency Response (H3)" {
          n72 = Divide(x=w165, y=w164) -> (x/y=w167:cdb[])
        }
      }
      n73 = Divide(x=w142, y=w141) -> (x/y=w146:dbl[])
      n74 = Bundle By Name(cluster=cluster{"f0":dbl, "df":dbl, "coherence":dbl[]} {"f0"=0.0, "df"=0.0, "coherence"=[]} ("coherence"), "f0"=w135, "df"=w134, "coherence"=w146) -> (w152:cluster{"f0":dbl, "df":dbl, "coherence":dbl[]})
      n75 = call <vilib>:"svfa_Modify Enhanced Spectrum Info (Dual).vi"("spectrum info X"=w113, "spectrum info Y"=w136, "spectrum type"=w137) -> ("spectrum info"=w111:T3)  [unwired: 10 in, 2 out]
      n76 = call <vilib>:"svfa_Set Averaging Mode in Spectrum Info.vi"("averaging mode"=T11."Vector averaging", "spectrum info in"=w111) -> ("spectrum info out"=w110:T3)  [unwired: 8 in, 1 out]
      n77 = Bundle By Name(cluster=w122, "spectrum info"=w110, "complex spectrum response.complex spectrum"=w139) -> (w138:T9)
    }
  }
  "final conditions" <- w11
  "coherence" <- w10
  "average measurement spectrum out" <- w6
  "averages completed out" <- w1
